vi "Send Channel Configuration (SubVI).vi"(8 "error in":errorcluster, 11 "Operation Index":i32) -> (0 "error out":errorcluster, 3 "Command Data":string[](array[string]))   [LabVIEW 2024]
uses:
  Digital Output/SubVIs/Digital Dynamic Cluster.ctl
  Analog Output/Controls/AO JSON Data Cluster.ctl
  Analog Output/Controls/AO Interface Data Cluster.ctl
  Analog Output/Controls/AO Channel Configuration Cluster.ctl
  Analog Output/Controls/AO Timing Cluster.ctl
  Digital Output/Controls/DIO Configuration cluster.ctl
  Digital Output/Controls/DIO Interface Data.ctl
  Async JSON Cluster.ctl
  Async Interface Data Cluster.ctl
  Async Serial/Controls/Async Serial Configuration Cluster.ctl
  Async Serial/Controls/Async Frame Info Cluster.ctl
  Async Serial/Controls/Async Message Info Cluster.ctl
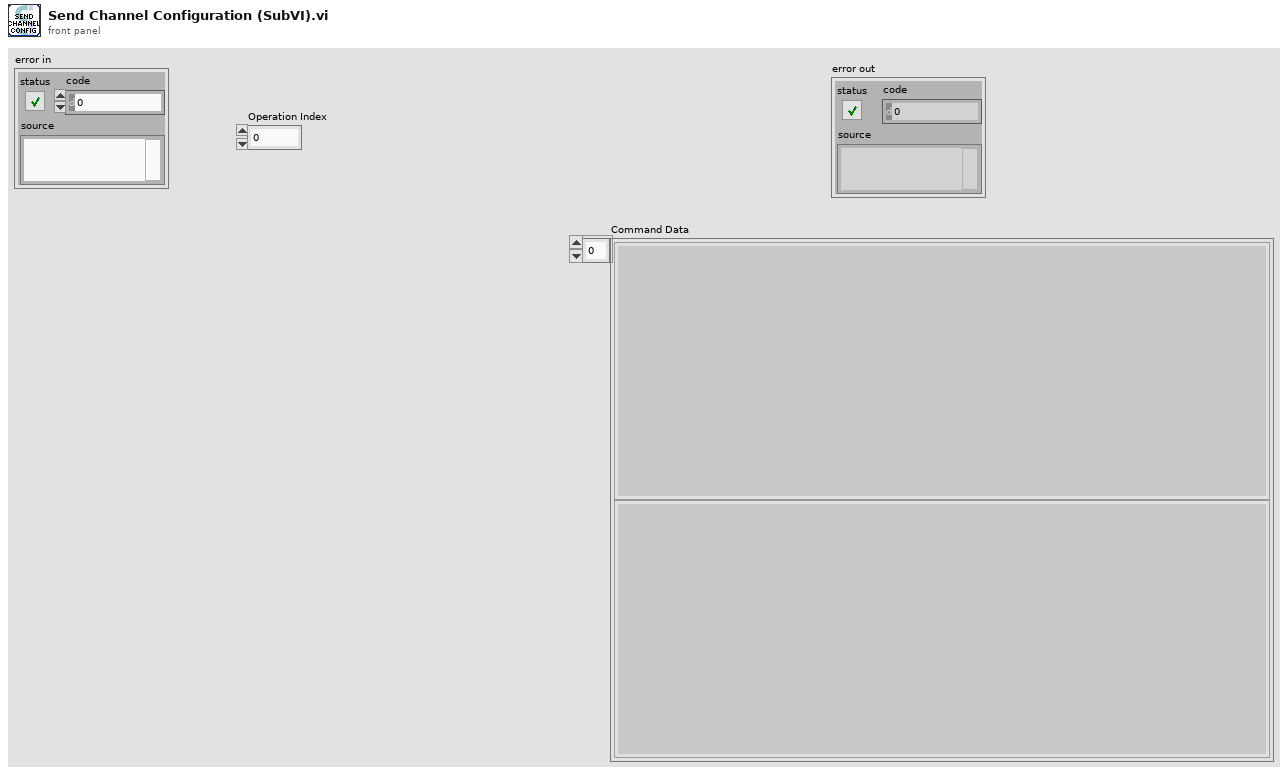
[diagram p1: front panel]
types:
  T1 = typedef "AO JSON Data Cluster.ctl" = cluster{"Interface":string, "Interface Data":T2}
  T2 = typedef "AO Interface Data Cluster.ctl" = cluster{"Command":string, "SubCmd":string, "Data":T3[], "Timing":T4}
  T3 = typedef "AO Channel Configuration Cluster.ctl" = cluster{"Channel":string, "Min Value":dbl, "Max Value":dbl, "Type":string, "Terminal Configure":u16, "Dynamic":u8, "Dyn Type":string, "Data":dbl[], "File Name":string, "Column":i32, "Frequency":dbl}
  T4 = typedef "AO Timing Cluster.ctl" = cluster{"samples per channel":i32, "sample mode":i32, "Sampling Rate":dbl}
  T5 = typedef "DIO Configuration cluster.ctl" = cluster{"Interface":string, "Interface Data":T6}
  T6 = typedef "DIO Interface Data.ctl" = cluster{"Command":string, "SubCmd":string, "Frequency":u16, "Data":T7[]}
  T7 = typedef "Digital Dynamic Cluster.ctl" = cluster{"Channel":string, "Data":u8[], "Identification Name":string}
  T8 = typedef "Async JSON Cluster.ctl" = cluster{"Interface":string, "Interface Data":T9}
  T9 = typedef "Async Interface Data Cluster.ctl" = cluster{"Command":string, "SubCmd":string, "Data":T10[]}
  T10 = typedef "Async Serial Configuration Cluster.ctl" = cluster{"Port":string, "Minor Frame Freq":u16, "Minor Frame Count":u16, "Frame Info":T11[], "Sensor Type":u16, "OIM Address":u16}
  T11 = typedef "Async Frame Info Cluster.ctl" = cluster{"Frame ID":u16, "Message Info":T12[]}
  T12 = typedef "Async Message Info Cluster.ctl" = cluster{"Message":u8[], "Message Name":string}
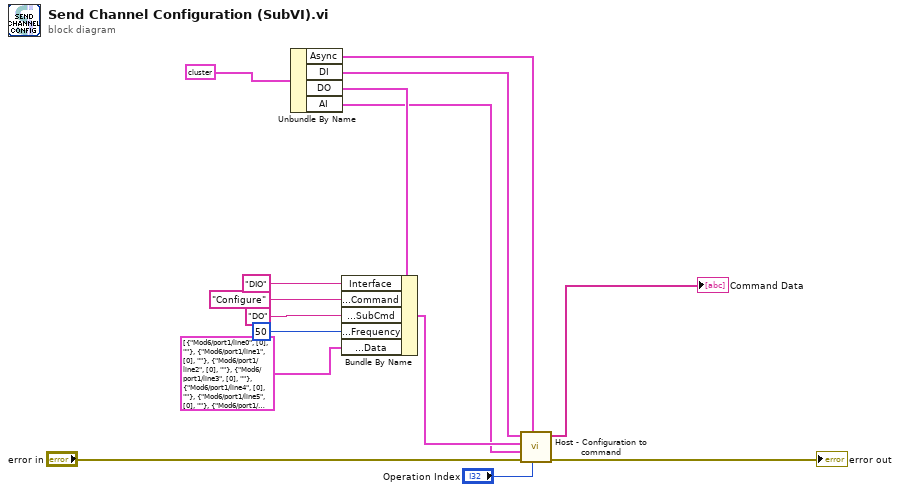
[diagram p0: block diagram]
diagram:
  n1 = Unbundle By Name(cluster{"AI":T1, "DI":T5, "DO":T5, "Async":T8} {"AI"={"Interface"="AIO", "Interface Data"={"Command"="Configure", "SubCmd"="AI", "Data"=[{"Channel"="Mod2/ai0", "Min Value"=-5.0, "Max Value"=5.0, "Type"="Voltage", "Terminal Configure"=10083, "Dynamic"=0, "Dyn Type"="", "Data"=[], "File Name"="", "Column"=0, "Frequency"=0.0}, {"Channel"="Mod2/ai1", "Min Value"=-5.0, "Max Value"=5.0, "Type"="Voltage", "Terminal Configure"=10083, "Dynamic"=0, "Dyn Type"="", "Data"=[], "File Name"="", "Column"=0, "Frequency"=0.0}, {"Channel"="Mod2/ai2", "Min Value"=-5.0, "Max Value"=5.0, "Type"="Voltage", "Terminal Configure"=10083, "Dynamic"=0, "Dyn Type"="", "Data"=[], "File Name"="", "Column"=0, "Frequency"=0.0}, {"Channel"="Mod2/ai3", "Min Value"=-5.0, "Max Value"=5.0, "Type"="Voltage", "Terminal Configure"=10083, "Dynamic"=0, "Dyn Type"="", "Data"=[], "File Name"="", "Column"=0, "Frequency"=0.0}, {"Channel"="Mod2/ai4", "Min Value"=-5.0, "Max Value"=5.0, "Type"="Voltage", "Terminal Configure"=10083, "Dynamic"=0, "Dyn Type"="", "Data"=[], "File Name"="", "Column"=0, "Frequency"=0.0}, {"Channel"="Mod2/ai5", "Min Value"=-5.0, "Max Value"=5.0, "Type"="Voltage", "Terminal Configure"=10083, "Dynamic"=0, "Dyn Type"="", "Data"=[], "File Name"="", "Column"=0, "Frequency"=0.0}, {"Channel"="Mod2/ai6", "Min Value"=-5.0, "Max Value"=5.0, "Type"="Voltage", "Terminal Configure"=10083, "Dynamic"=0, "Dyn Type"="", "Data"=[], "File Name"="", "Column"=0, "Frequency"=0.0}, {"Channel"="Mod2/ai7", "Min Value"=-5.0, "Max Value"=5.0, "Type"="Voltage", "Terminal Configure"=10083, "Dynamic"=0, "Dyn Type"="", "Data"=[], "File Name"="", "Column"=0, "Frequency"=0.0}, {"Channel"="Mod2/ai8", "Min Value"=-5.0, "Max Value"=5.0, "Type"="Voltage", "Terminal Configure"=10083, "Dynamic"=0, "Dyn Type"="", "Data"=[], "File Name"="", "Column"=0, "Frequency"=0.0}, {"Channel"="Mod2/ai9", "Min Value"=-5.0, "Max Value"=5.0, "Type"="Voltage", "Terminal Configure"=10083, "Dynamic"=0, "Dyn Type"="", "Data"=[], "File Name"="", "Column"=0, "Frequency"=0.0}, {"Channel"="Mod2/ai10", "Min Value"=-5.0, "Max Value"=5.0, "Type"="Voltage", "Terminal Configure"=10083, "Dynamic"=0, "Dyn Type"="", "Data"=[], "File Name"="", "Column"=0, "Frequency"=0.0}, {"Channel"="Mod2/ai11", "Min Value"=-5.0, "Max Value"=5.0, "Type"="Voltage", "Terminal Configure"=10083, "Dynamic"=0, "Dyn Type"="", "Data"=[], "File Name"="", "Column"=0, "Frequency"=0.0}, {"Channel"="Mod2/ai12", "Min Value"=-5.0, "Max Value"=5.0, "Type"="Voltage", "Terminal Configure"=10083, "Dynamic"=0, "Dyn Type"="", "Data"=[], "File Name"="", "Column"=0, "Frequency"=0.0}, {"Channel"="Mod2/ai13", "Min Value"=-5.0, "Max Value"=5.0, "Type"="Voltage", "Terminal Configure"=10083, "Dynamic"=0, "Dyn Type"="", "Data"=[], "File Name"="", "Column"=0, "Frequency"=0.0}, {"Channel"="Mod2/ai14", "Min Value"=-5.0, "Max Value"=5.0, "Type"="Voltage", "Terminal Configure"=10083, "Dynamic"=0, "Dyn Type"="", "Data"=[], "File Name"="", "Column"=0, "Frequency"=0.0}, {"Channel"="Mod2/ai15", "Min Value"=-5.0, "Max Value"=5.0, "Type"="Voltage", "Terminal Configure"=10083, "Dynamic"=0, "Dyn Type"="", "Data"=[], "File Name"="", "Column"=0, "Frequency"=0.0}, {"Channel"="Mod2/ai16", "Min Value"=-5.0, "Max Value"=5.0, "Type"="Voltage", "Terminal Configure"=10083, "Dynamic"=0, "Dyn Type"="", "Data"=[], "File Name"="", "Column"=0, "Frequency"=0.0}, {"Channel"="Mod2/ai17", "Min Value"=-5.0, "Max Value"=5.0, "Type"="Voltage", "Terminal Configure"=10083, "Dynamic"=0, "Dyn Type"="", "Data"=[], "File Name"="", "Column"=0, "Frequency"=0.0}, {"Channel"="Mod2/ai18", "Min Value"=-5.0, "Max Value"=5.0, "Type"="Voltage", "Terminal Configure"=10083, "Dynamic"=0, "Dyn Type"="", "Data"=[], "File Name"="", "Column"=0, "Frequency"=0.0}, {"Channel"="Mod2/ai19", "Min Value"=-5.0, "Max Value"=5.0, "Type"="Voltage", "Terminal Configure"=10083, "Dynamic"=0, "Dyn Type"="", "Data"=[], "File Name"="", "Column"=0, "Frequency"=0.0}, {"Channel"="Mod2/ai20", "Min Value"=-5.0, "Max Value"=5.0, "Type"="Voltage", "Terminal Configure"=10083, "Dynamic"=0, "Dyn Type"="", "Data"=[], "File Name"="", "Column"=0, "Frequency"=0.0}, {"Channel"="Mod2/ai21", "Min Value"=-5.0, "Max Value"=5.0, "Type"="Voltage", "Terminal Configure"=10083, "Dynamic"=0, "Dyn Type"="", "Data"=[], "File Name"="", "Column"=0, "Frequency"=0.0}, {"Channel"="Mod2/ai22", "Min Value"=-5.0, "Max Value"=5.0, "Type"="Voltage", "Terminal Configure"=10083, "Dynamic"=0, "Dyn Type"="", "Data"=[], "File Name"="", "Column"=0, "Frequency"=0.0}, {"Channel"="Mod2/ai23", "Min Value"=-5.0, "Max Value"=5.0, "Type"="Voltage", "Terminal Configure"=10083, "Dynamic"=0, "Dyn Type"="", "Data"=[], "File Name"="", "Column"=0, "Frequency"=0.0}, {"Channel"="Mod2/ai24", "Min Value"=-5.0, "Max Value"=5.0, "Type"="Voltage", "Terminal Configure"=10083, "Dynamic"=0, "Dyn Type"="", "Data"=[], "File Name"="", "Column"=0, "Frequency"=0.0}, {"Channel"="Mod2/ai25", "Min Value"=-5.0, "Max Value"=5.0, "Type"="Voltage", "Terminal Configure"=10083, "Dynamic"=0, "Dyn Type"="", "Data"=[], "File Name"="", "Column"=0, "Frequency"=0.0}, {"Channel"="Mod2/ai26", "Min Value"=-5.0, "Max Value"=5.0, "Type"="Voltage", "Terminal Configure"=10083, "Dynamic"=0, "Dyn Type"="", "Data"=[], "File Name"="", "Column"=0, "Frequency"=0.0}, {"Channel"="Mod2/ai27", "Min Value"=-5.0, "Max Value"=5.0, "Type"="Voltage", "Terminal Configure"=10083, "Dynamic"=0, "Dyn Type"="", "Data"=[], "File Name"="", "Column"=0, "Frequency"=0.0}, {"Channel"="Mod2/ai28", "Min Value"=-5.0, "Max Value"=5.0, "Type"="Voltage", "Terminal Configure"=10083, "Dynamic"=0, "Dyn Type"="", "Data"=[], "File Name"="", "Column"=0, "Frequency"=0.0}, {"Channel"="Mod2/ai29", "Min Value"=-5.0, "Max Value"=5.0, "Type"="Voltage", "Terminal Configure"=10083, "Dynamic"=0, "Dyn Type"="", "Data"=[], "File Name"="", "Column"=0, "Frequency"=0.0}, {"Channel"="Mod2/ai30", "Min Value"=-5.0, "Max Value"=5.0, "Type"="Voltage", "Terminal Configure"=10083, "Dynamic"=0, "Dyn Type"="", "Data"=[], "File Name"="", "Column"=0, "Frequency"=0.0}, {"Channel"="Mod2/ai31", "Min Value"=-5.0, "Max Value"=5.0, "Type"="Voltage", "Terminal Configure"=65535, "Dynamic"=0, "Dyn Type"="", "Data"=[], "File Name"="", "Column"=0, "Frequency"=0.0}], "Timing"={"samples per channel"=4, "sample mode"=10123, "Sampling Rate"=2.0}}}, "DI"={"Interface"="DIO", "Interface Data"={"Command"="Configure", "SubCmd"="DI", "Frequency"=500, "Data"=[{"Channel"="Mod3/port0/line0", "Data"=[0], "Identification Name"=""}, {"Channel"="Mod3/port0/line1", "Data"=[0], "Identification Name"=""}, {"Channel"="Mod3/port0/line2", "Data"=[0], "Identification Name"=""}, {"Channel"="Mod3/port0/line3", "Data"=[0], "Identification Name"=""}, {"Channel"="Mod3/port0/line4", "Data"=[0], "Identification Name"=""}, {"Channel"="Mod3/port0/line5", "Data"=[0], "Identification Name"=""}, {"Channel"="Mod3/port0/line6", "Data"=[0], "Identification Name"=""}, {"Channel"="Mod3/port0/line7", "Data"=[0], "Identification Name"=""}, {"Channel"="Mod3/port0/line8", "Data"=[0], "Identification Name"=""}, {"Channel"="Mod3/port0/line9", "Data"=[0], "Identification Name"=""}, {"Channel"="Mod3/port0/line10", "Data"=[0], "Identification Name"=""}, {"Channel"="Mod3/port0/line11", "Data"=[0], "Identification Name"=""}, {"Channel"="Mod3/port0/line12", "Data"=[0], "Identification Name"=""}, {"Channel"="Mod3/port0/line13", "Data"=[0], "Identification Name"=""}, {"Channel"="Mod3/port0/line14", "Data"=[0], "Identification Name"=""}, {"Channel"="Mod3/port0/line15", "Data"=[0], "Identification Name"=""}, {"Channel"="Mod3/port0/line16", "Data"=[0], "Identification Name"=""}, {"Channel"="Mod3/port0/line17", "Data"=[0], "Identification Name"=""}, {"Channel"="Mod3/port0/line18", "Data"=[0], "Identification Name"=""}, {"Channel"="Mod3/port0/line19", "Data"=[0], "Identification Name"=""}, {"Channel"="Mod3/port0/line20", "Data"=[0], "Identification Name"=""}, {"Channel"="Mod3/port0/line21", "Data"=[0], "Identification Name"=""}, {"Channel"="Mod3/port0/line22", "Data"=[0], "Identification Name"=""}, {"Channel"="Mod3/port0/line23", "Data"=[0], "Identification Name"=""}, {"Channel"="Mod3/port0/line24", "Data"=[0], "Identification Name"=""}, {"Channel"="Mod3/port0/line25", "Data"=[0], "Identification Name"=""}, {"Channel"="Mod3/port0/line26", "Data"=[0], "Identification Name"=""}, {"Channel"="Mod3/port0/line27", "Data"=[0], "Identification Name"=""}, {"Channel"="Mod3/port0/line28", "Data"=[0], "Identification Name"=""}, {"Channel"="Mod3/port0/line29", "Data"=[0], "Identification Name"=""}, {"Channel"="Mod3/port0/line30", "Data"=[0], "Identification Name"=""}, {"Channel"="Mod3/port0/line31", "Data"=[0], "Identification Name"=""}, {"Channel"="Mod4/port0/line0", "Data"=[0], "Identification Name"=""}, {"Channel"="Mod4/port0/line1", "Data"=[0], "Identification Name"=""}, {"Channel"="Mod4/port0/line2", "Data"=[0], "Identification Name"=""}, {"Channel"="Mod4/port0/line3", "Data"=[0], "Identification Name"=""}, {"Channel"="Mod4/port0/line4", "Data"=[0], "Identification Name"=""}, {"Channel"="Mod4/port0/line5", "Data"=[0], "Identification Name"=""}, {"Channel"="Mod4/port0/line6", "Data"=[0], "Identification Name"=""}, {"Channel"="Mod4/port0/line7", "Data"=[0], "Identification Name"=""}, {"Channel"="Mod4/port0/line8", "Data"=[0], "Identification Name"=""}, {"Channel"="Mod4/port0/line9", "Data"=[0], "Identification Name"=""}, {"Channel"="Mod4/port0/line10", "Data"=[0], "Identification Name"=""}, {"Channel"="Mod4/port0/line11", "Data"=[0], "Identification Name"=""}, {"Channel"="Mod4/port0/line12", "Data"=[0], "Identification Name"=""}, {"Channel"="Mod4/port0/line13", "Data"=[0], "Identification Name"=""}, {"Channel"="Mod4/port0/line14", "Data"=[0], "Identification Name"=""}, {"Channel"="Mod4/port0/line15", "Data"=[0], "Identification Name"=""}, {"Channel"="Mod4/port0/line16", "Data"=[0], "Identification Name"=""}, {"Channel"="Mod4/port0/line17", "Data"=[0], "Identification Name"=""}, {"Channel"="Mod4/port0/line18", "Data"=[0], "Identification Name"=""}, {"Channel"="Mod4/port0/line19", "Data"=[0], "Identification Name"=""}, {"Channel"="Mod4/port0/line20", "Data"=[0], "Identification Name"=""}, {"Channel"="Mod4/port0/line21", "Data"=[0], "Identification Name"=""}, {"Channel"="Mod4/port0/line22", "Data"=[0], "Identification Name"=""}, {"Channel"="Mod4/port0/line23", "Data"=[0], "Identification Name"=""}, {"Channel"="Mod4/port0/line24", "Data"=[0], "Identification Name"=""}, {"Channel"="Mod4/port0/line25", "Data"=[0], "Identification Name"=""}, {"Channel"="Mod4/port0/line26", "Data"=[0], "Identification Name"=""}, {"Channel"="Mod4/port0/line27", "Data"=[0], "Identification Name"=""}, {"Channel"="Mod4/port0/line28", "Data"=[0], "Identification Name"=""}, {"Channel"="Mod4/port0/line29", "Data"=[0], "Identification Name"=""}, {"Channel"="Mod4/port0/line30", "Data"=[0], "Identification Name"=""}, {"Channel"="Mod4/port0/line31", "Data"=[0], "Identification Name"=""}]}}, "DO"={"Interface"="DIO", "Interface Data"={"Command"="Configure", "SubCmd"="DO", "Frequency"=500, "Data"=[{"Channel"="Mod1/port0/line0", "Data"=[0], "Identification Name"=""}, {"Channel"="Mod1/port0/line1", "Data"=[0], "Identification Name"=""}, {"Channel"="Mod1/port0/line2", "Data"=[0], "Identification Name"=""}, {"Channel"="Mod1/port0/line3", "Data"=[0], "Identification Name"=""}, {"Channel"="Mod1/port0/line4", "Data"=[0], "Identification Name"=""}, {"Channel"="Mod1/port0/line5", "Data"=[0], "Identification Name"=""}, {"Channel"="Mod1/port0/line6", "Data"=[0], "Identification Name"=""}, {"Channel"="Mod1/port0/line7", "Data"=[0], "Identification Name"=""}, {"Channel"="Mod1/port0/line8", "Data"=[0], "Identification Name"=""}, {"Channel"="Mod1/port0/line9", "Data"=[0], "Identification Name"=""}, {"Channel"="Mod1/port0/line10", "Data"=[0], "Identification Name"=""}, {"Channel"="Mod1/port0/line11", "Data"=[0], "Identification Name"=""}, {"Channel"="Mod1/port0/line12", "Data"=[0], "Identification Name"=""}, {"Channel"="Mod1/port0/line13", "Data"=[0], "Identification Name"=""}, {"Channel"="Mod1/port0/line14", "Data"=[0], "Identification Name"=""}, {"Channel"="Mod1/port0/line15", "Data"=[0], "Identification Name"=""}, {"Channel"="Mod1/port0/line16", "Data"=[0], "Identification Name"=""}, {"Channel"="Mod1/port0/line17", "Data"=[0], "Identification Name"=""}, {"Channel"="Mod1/port0/line18", "Data"=[0], "Identification Name"=""}, {"Channel"="Mod1/port0/line19", "Data"=[0], "Identification Name"=""}, {"Channel"="Mod1/port0/line20", "Data"=[0], "Identification Name"=""}, {"Channel"="Mod1/port0/line21", "Data"=[0], "Identification Name"=""}, {"Channel"="Mod1/port0/line22", "Data"=[0], "Identification Name"=""}, {"Channel"="Mod1/port0/line23", "Data"=[0], "Identification Name"=""}, {"Channel"="Mod1/port0/line24", "Data"=[0], "Identification Name"=""}, {"Channel"="Mod1/port0/line25", "Data"=[0], "Identification Name"=""}, {"Channel"="Mod1/port0/line26", "Data"=[0], "Identification Name"=""}, {"Channel"="Mod1/port0/line27", "Data"=[0], "Identification Name"=""}, {"Channel"="Mod1/port0/line28", "Data"=[0], "Identification Name"=""}, {"Channel"="Mod1/port0/line29", "Data"=[0], "Identification Name"=""}, {"Channel"="Mod1/port0/line30", "Data"=[0], "Identification Name"=""}, {"Channel"="Mod1/port0/line31", "Data"=[0], "Identification Name"=""}]}}, "Async"={"Interface"="Async", "Interface Data"={"Command"="Configure", "SubCmd"="Async", "Data"=[{"Port"="com10", "Minor Frame Freq"=200, "Minor Frame Count"=1, "Frame Info"=[{"Frame ID"=1, "Message Info"=[{"Message"=[1], "Message Name"="m1"}]}], "Sensor Type"=0, "OIM Address"=0}]}}} ("Channel Data")) -> ("Async"=w9:T8, "DI"=w10:T5, "DO"=w2:T5, "AI"=w1:T1)
  n2 = Bundle By Name(cluster=w2, "Interface"="DIO" ("DO.Interface"), "Interface Data.Command"="Configure" ("DO.Interface Data.Command"), "Interface Data.SubCmd"="DO" ("DO.Interface Data.SubCmd"), "Interface Data.Frequency"=u16 50 ("DO.Interface Data.Frequency"), "Interface Data.Data"=T7[] [{"Channel"="Mod6/port1/line0", "Data"=[0], "Identification Name"=""}, {"Channel"="Mod6/port1/line1", "Data"=[0], "Identification Name"=""}, {"Channel"="Mod6/port1/line2", "Data"=[0], "Identification Name"=""}, {"Channel"="Mod6/port1/line3", "Data"=[0], "Identification Name"=""}, {"Channel"="Mod6/port1/line4", "Data"=[0], "Identification Name"=""}, {"Channel"="Mod6/port1/line5", "Data"=[0], "Identification Name"=""}, {"Channel"="Mod6/port1/line6", "Data"=[0], "Identification Name"=""}, {"Channel"="Mod6/port1/line7", "Data"=[0], "Identification Name"=""}, {"Channel"="Mod6/port1/line8", "Data"=[0], "Identification Name"=""}, {"Channel"="Mod6/port1/line9", "Data"=[0], "Identification Name"=""}, {"Channel"="Mod6/port1/line10", "Data"=[0], "Identification Name"=""}, {"Channel"="Mod6/port1/line11", "Data"=[0], "Identification Name"=""}, {"Channel"="Mod6/port1/line12", "Data"=[0], "Identification Name"=""}, {"Channel"="Mod6/port1/line13", "Data"=[0], "Identification Name"=""}, {"Channel"="Mod6/port1/line14", "Data"=[0], "Identification Name"=""}, {"Channel"="Mod6/port1/line15", "Data"=[0], "Identification Name"=""}] ("DO.Interface Data.Data")) -> (w3:T5)
  n3 = call "Host - Configuration to command.vi"("Operation Index"="Operation Index", "Async"=w9, "error in"="error in", "AI"=w1, "DO"=w3, "DI"=w10) -> ("error out"=→"error out":errorcluster, "Command Data"=→"Command Data":string[])  [unwired: 4 in]
